vi "etlWriteDynReg.vi"() -> ()   [LabVIEW 2017]
uses:
  <vilib>/DAQmx/write.llb/DAQmx Write (Analog 2D DBL NChan NSamp).vi
  globalDevices.vi
  globalUtilities.vi
  <vilib>/DAQmx/miscellaneous.llb/DAQmx Fill In Error Info.vi
panel:
  out "success":bool
  out "Waveform Graph 3":dbl[](graph)
  out "nT":i32
  out "dt":dbl
  out "omega":dbl
  out "amplitude":dbl
  out "offset":dbl
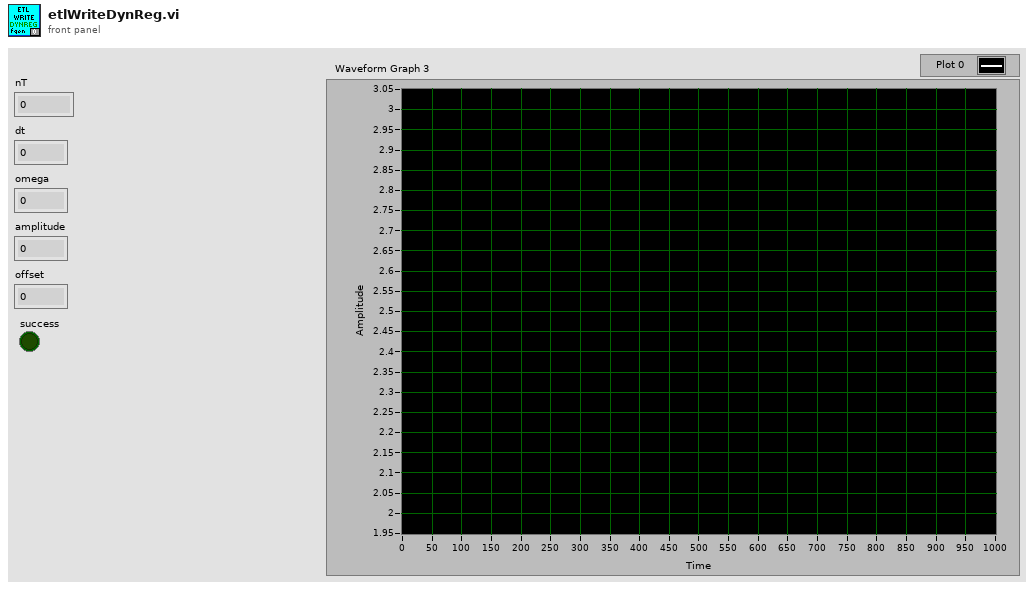
[diagram p1: front panel]
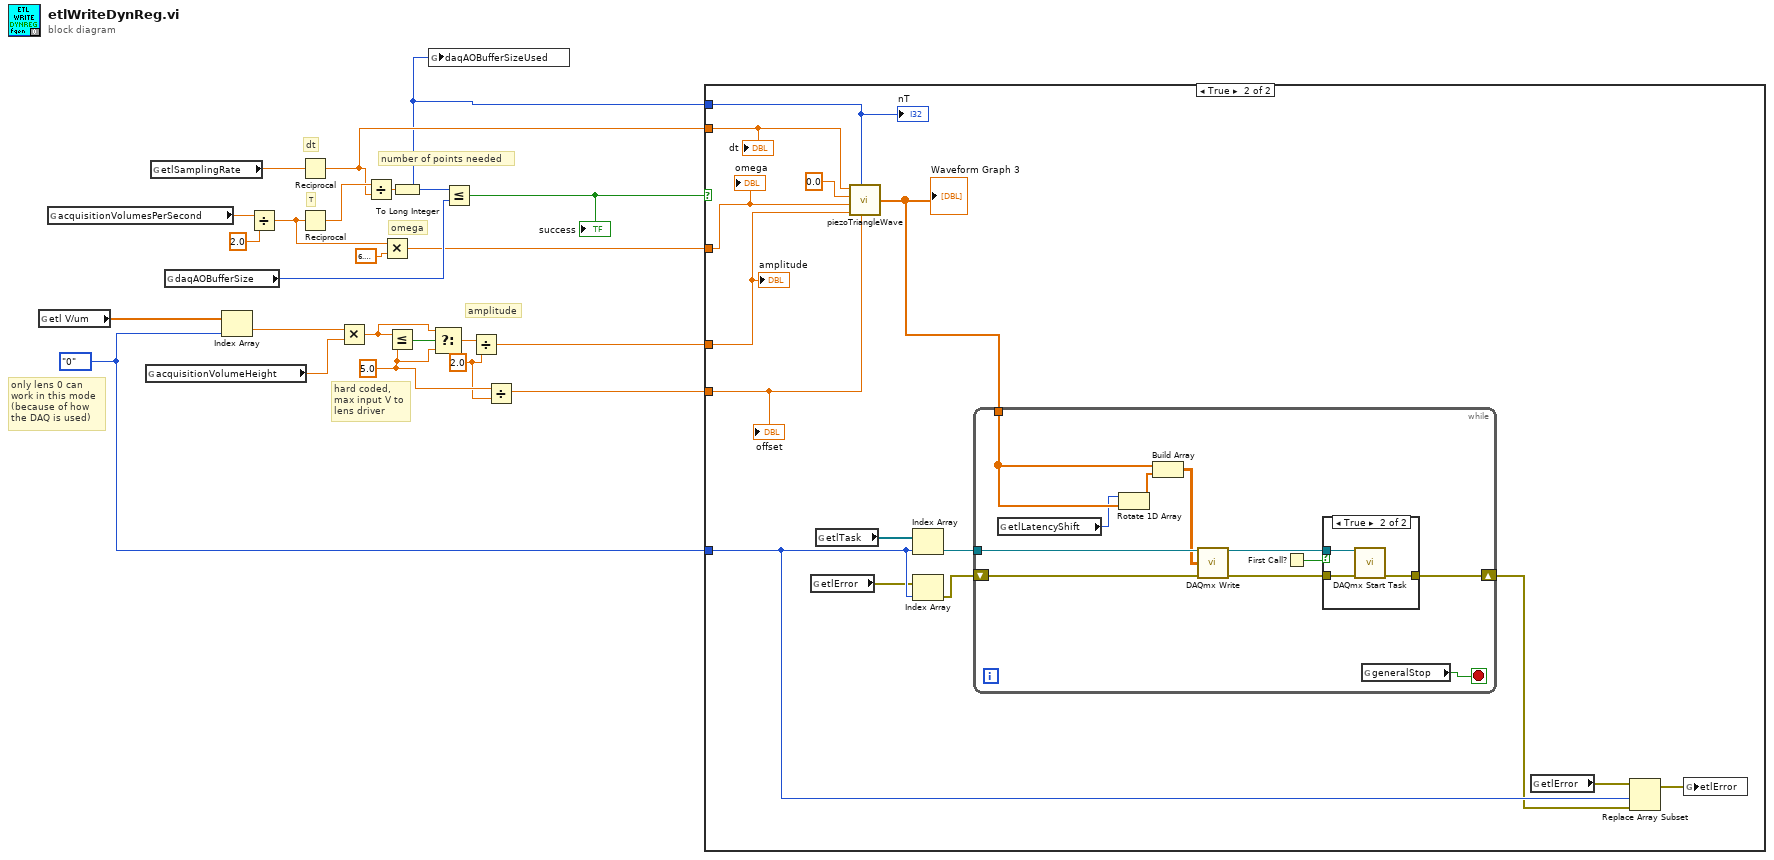
[diagram p0: block diagram]
diagram:
  w1 = enum16{"0", "1"}."0" ("lens")
  w4 = 5.0 ("y")
  w3 = 2.0 ("y")
  # "only lens 0 can\nwork in this mode\n(because of how\nthe DAQ is used)"
  # "hard coded,\nmax input V to\nlens driver"
  # "omega"
  # "amplitude"
  # "number of points needed"
  # "T"
  # "dt"
  n1 = global read "globalDevices.vi" "etl V/um"() -> (w6:dbl[])
  n2 = global read "globalUtilities.vi" "acquisitionVolumesPerSecond"() -> (w22:dbl)
  n3 = global read "globalUtilities.vi" "acquisitionVolumeHeight"() -> (w17:dbl)
  n4 = global read "globalDevices.vi" "etlSamplingRate"() -> (w23:dbl)
  n5 = global read "globalDevices.vi" "daqAOBufferSize"() -> (w19:i32)
  n6 = Index Array(array=w6, index=w1) -> (element=w5:dbl)
  n7 = Divide(x=w22, y=2.0) -> (x/y=w11:dbl)
  n8 = Reciprocal(x=w23) -> (1/x=w9:dbl)
  n9 = Reciprocal(x=w11) -> (1/x=w20:dbl)
  n10 = Multiply(x=w5, y=w17) -> (x*y=w15:dbl)
  n11 = Divide(x=w20, y=w9) -> (x/y=w8:dbl)
  n12 = Multiply(x=w11, y=6.283185307179586) -> (x*y=w10:dbl)
  n13 = Less Or Equal?(x=w15, y=w4) -> (x <= y?=w16:bool)
  n14 = To Long Integer(number=w8) -> (32bit integer=w7:i32)
  n15 = global write "globalDevices.vi" "daqAOBufferSizeUsed"(w7) -> ()
  n16 = Select(t=w15, s=w16, f=w4) -> (s? t:f=w14:dbl)
  n17 = Less Or Equal?(x=w7, y=w19) -> (x <= y?=w18:bool)
  "success" <- w18
  n18 = Divide(x=w14, y=w3) -> (x/y=w13:dbl)
  n19 = Divide(x=w4, y=w3) -> (x/y=w2:dbl)
  n20 = case shown="True" w18 {
    tunnel: w13 -> [_ w34]
    tunnel: w2 -> [_ w33]
    tunnel: w10 -> [_ w35]
    tunnel: w7 -> [_ w37]
    tunnel: w9 -> [_ w36]
    tunnel: w1 -> [_ w32]
    frame False {
    }
    frame True {
      n21 = global read "globalDevices.vi" "etlError"() -> (w29:errorcluster[])
      n22 = global read "globalDevices.vi" "etlTask"() -> (w30:refnum<k21>[])
      n23 = call "piezoTriangleWave.vi"("offset"=w33, "nT"=w37, "amplitude"=w34, "omega"=w35, "t0"=0.0, "dt"=w36) -> ("x+y"=w31:dbl[])
      "Waveform Graph 3" <- w31
      n24 = Index Array(array=w30, index=w32) -> (element=w25:refnum<k21>)
      n25 = Index Array(array=w29, index=w32) -> (element=w24:errorcluster)
      n26 = while {
        tunnel: w31 -> [w41]
        tunnel: w25 -> [w46]
        shift-right: [w47] -> w27
        shift-left: w24 -> [w45]
        stop <- w43 stop-if-true
        n27 = global read "globalDevices.vi" "etlLatencyShift"() -> (w39:i8)
        n28 = Rotate 1D Array(1:w41, 2:w39) -> (0:w42:dbl[])
        n29 = Build Array(w41, w42) -> (w40:dbl[][])
        n30 = call-poly <vilib>:"DAQmx Write.vi"("task/channels in"=w46, "data"=w40, "error in"=w45) -> ("task out"=w48:refnum<k21>, "error out"=w49:errorcluster)  [unwired: 10 in, 1 out]
        n31 = First Call?() -> (First Call?: T/F=w44:bool)
        n32 = case shown="True" w44 {
          tunnel: w49 -> [w50 w53]
          tunnel: w48 -> [_ w52]
          tunnel: [w50 w51] -> w47
          frame False {
          }
          frame True {
            n33 = call <vilib>:"DAQmx Start Task.vi"("task/channels in"=w52, "error in"=w53) -> ("error out"=w51:errorcluster)  [unwired: 12 in, 1 out]
          }
        }
        n34 = global read "globalUtilities.vi" "generalStop"() -> (w43:bool)
      }
      n35 = global read "globalDevices.vi" "etlError"() -> (w28:errorcluster[])
      n36 = Replace Array Subset(array=w28, new element=w27, index=w32) -> (w26:errorcluster[])
      n37 = global write "globalDevices.vi" "etlError"(w26) -> ()
      "nT" <- w37
      "dt" <- w36
      "omega" <- w35
      "amplitude" <- w34
      "offset" <- w33
    }
  }
